vi "WriteRead Data.vi"(7 "SPI Peripheral":refnum<class "SPI Connection.lvclass">, 8 "error in (no error)":errorcluster, 10 "Write Data":string) -> (0 "error out":errorcluster, 1 "Read Data":string)   [LabVIEW 2020, in "CTI.lvlib" / "SPI Connection.lvclass"]
uses:
  SPI Connection.lvclass
  SPI Connection.lvclass/SPI Connection.ctl
  Session/Session.lvclass
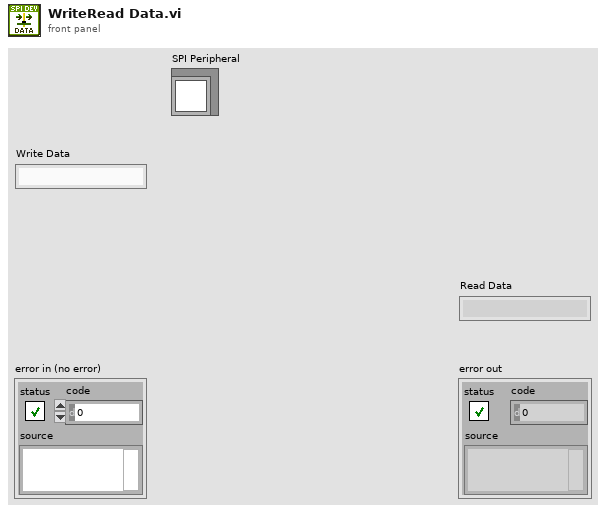
[diagram p1: front panel]
types:
  T1 = typedef "CTI.lvlib/SPI Number.ctl" = i8
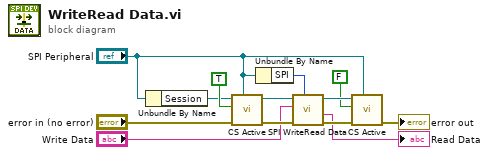
[diagram p0: block diagram]
diagram:
  n1 = Unbundle By Name("SPI Peripheral") -> ("Session"=w1:refnum<class "Session.lvclass">)
  n2 = call "CS Active.vi"("SPI Peripheral in"="SPI Peripheral", "error in (no error)"="error in (no error)", "CS Active"=TRUE, "Session In"=w1) -> ("error out"=w11:errorcluster, "Session Out"=w9:refnum<class "Session.lvclass">)  [unwired: 6 in]
  n3 = Unbundle By Name("SPI Peripheral") -> ("SPI"=w10:T1)
  n4 = call "SPI WriteRead Data.vi"("SPI #"=w10, "error in (no error)"=w11, "Write Data"="Write Data", "Session in"=w9) -> ("error out"=w12:errorcluster, "Read Data"=→"Read Data":string, "Session out"=w13:refnum<class "Session.lvclass">)  [unwired: 5 in]
  n5 = call "CS Active.vi"("SPI Peripheral in"="SPI Peripheral", "error in (no error)"=w12, "CS Active"=FALSE, "Session In"=w13) -> ("error out"=→"error out":errorcluster)  [unwired: 6 in, 1 out]
